vi "Code 0.0.5.vi"(0 "Value":refnum<k5>, 1 "status":bool, 2 "MaxSlide":dbl, 3 "File Path Control":path, 5 "Port":u16=8030, 7 "Connect Statut":refnum<vi>, 9 "Drv":u8(ring) items=["Drv 1", "Drv 2"], 11 "error in (no error)":errorcluster, 12 "Progress bar Value":refnum<vi>, 13 "String":refnum<vi>, 14 "Max":refnum<vi>) -> (4 "Error List":string, 6 "Status":bool, 15 "error out":errorcluster)   [LabVIEW 2017]
panel:
  out "Autobaud":bool
  in  "StopS.M. 2":bool
  in  "StopS.M.":bool
  in  "CatchNetworkFlag":bool
  in  "stop Listen":bool
  out "conn ID":refnum<k5>
  in  "Next Button":bool
  out "CheckSum":bool[][](array[boolean])
  out "CheckSum DataB":u16 format="%.0x"
  out "CheckSum Data":u16 format="%.0x"
  out "Writting Data":bool
  out "Send Header":bool
  out "sumHeader":u16 format="%.0x"
  # "Ver 0.0.7"
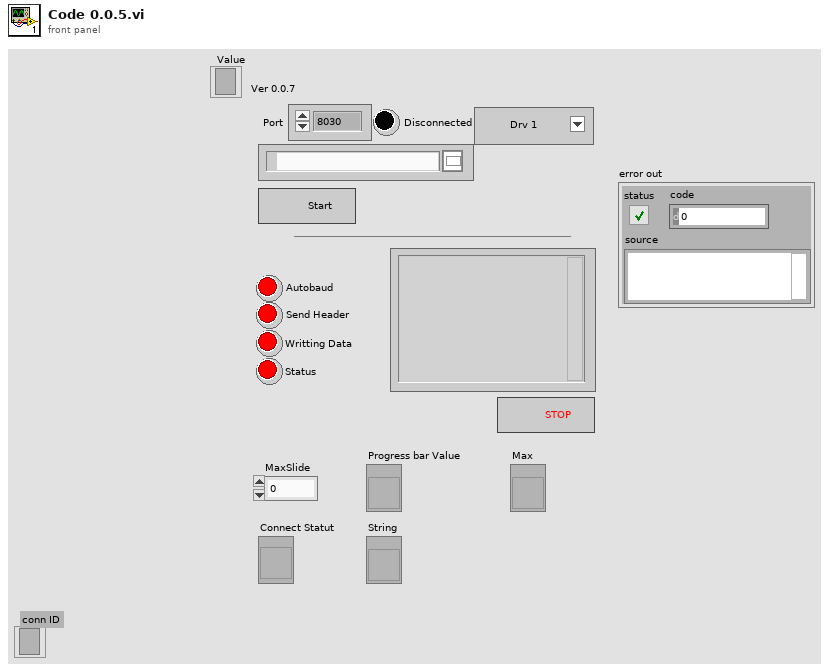
[diagram p1: front panel]
types:
  T1 = enum16{"open", "replace", "create", "open or create", "replace or create", "replace or create with confirmation"}
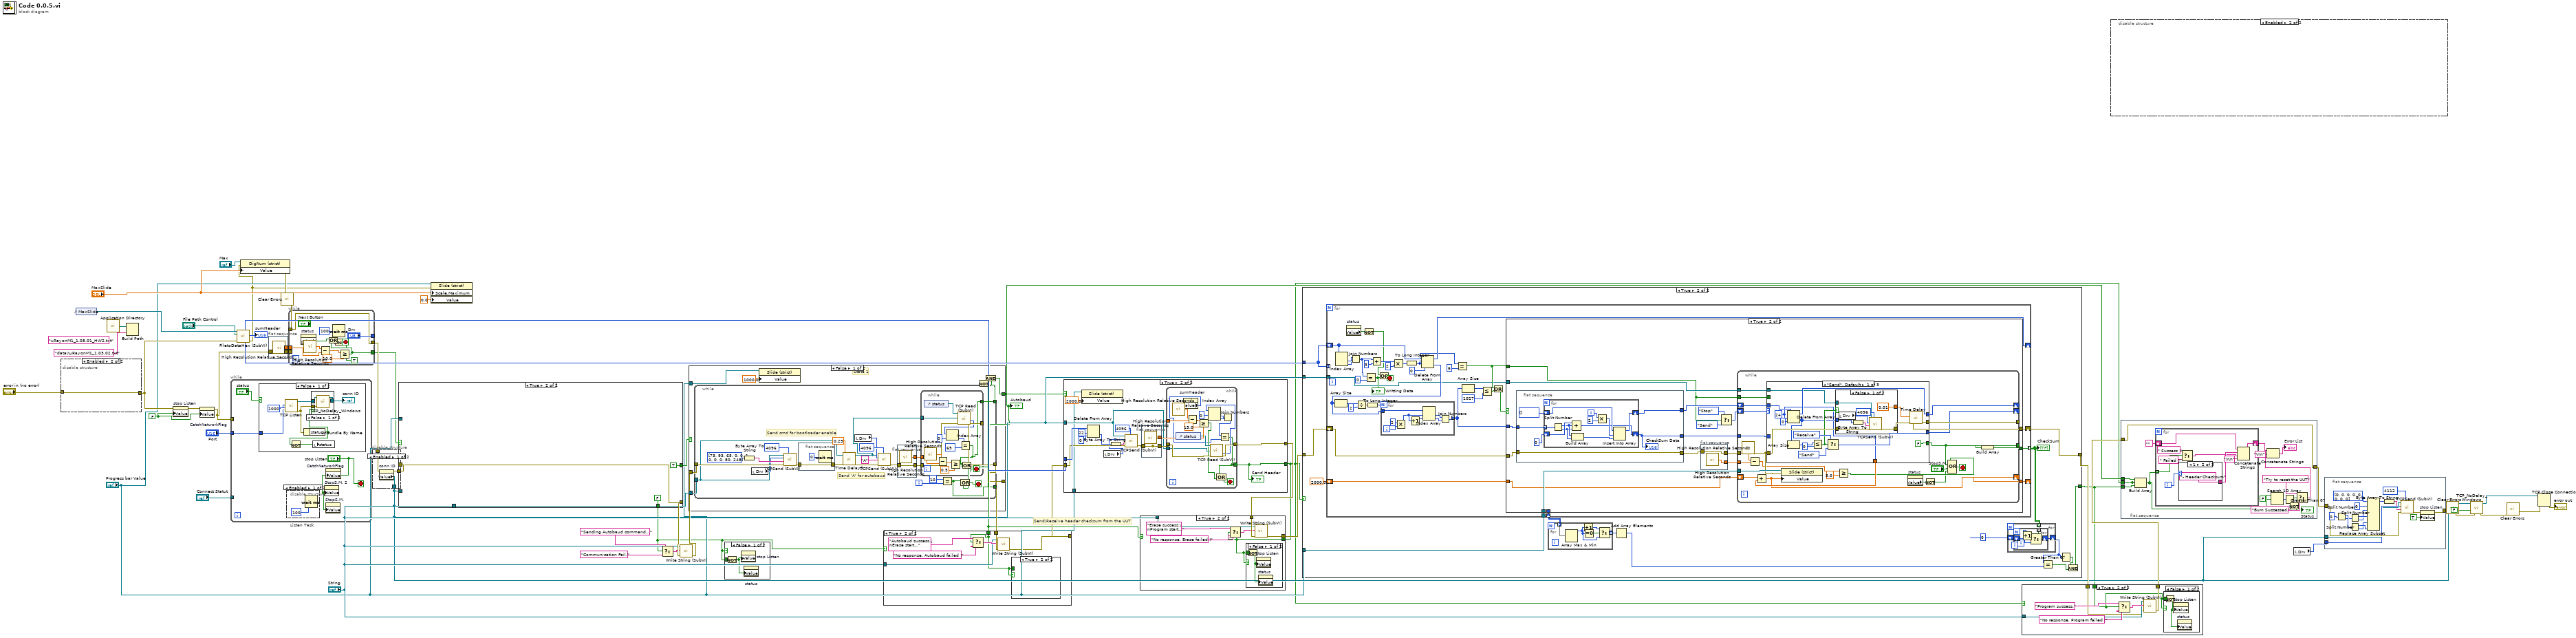
[diagram p0: block diagram]
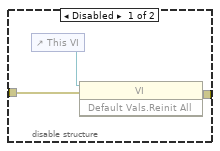
[diagram p2: hidden frame]
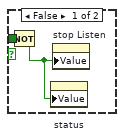
[diagram p7: hidden frame]
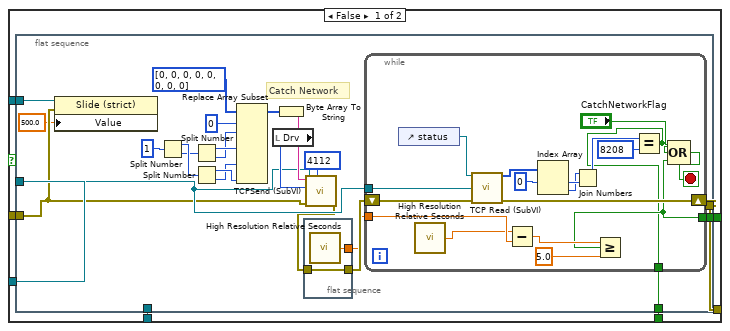
[diagram p10: hidden frame]
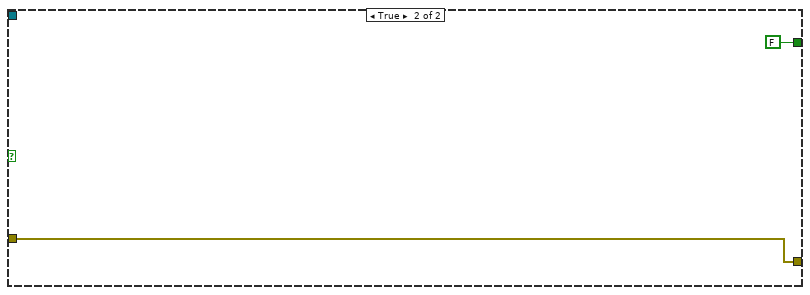
[diagram p11: hidden frame]
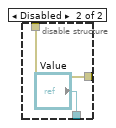
[diagram p12: hidden frame]
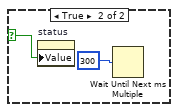
[diagram p15: hidden frame]
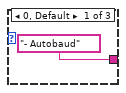
[diagram p16: hidden frame]
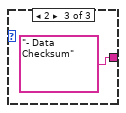
[diagram p17: hidden frame]
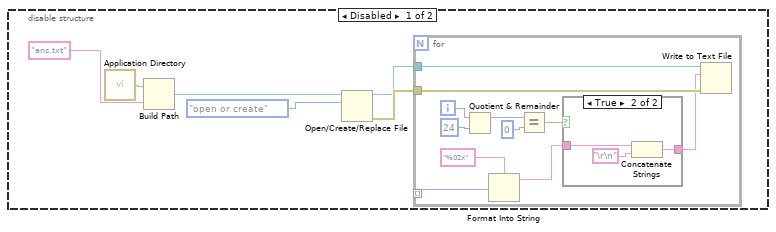
[diagram p18: hidden frame]
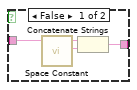
[diagram p19: hidden frame]
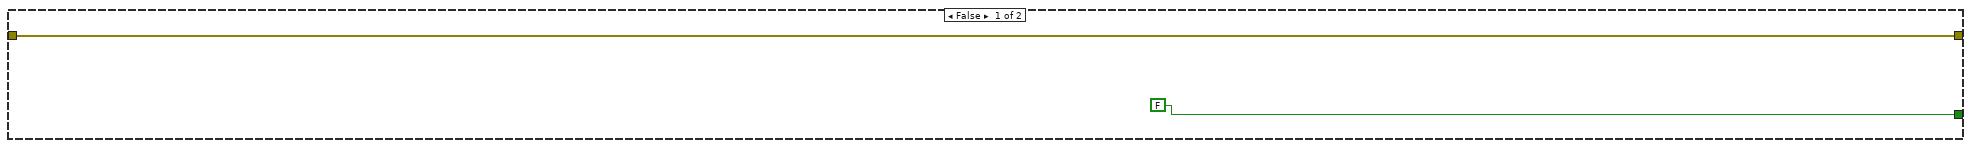
[diagram p20: hidden frame]
diagram:
  (unwired) "uRayonM1_1.05.01_HW2.txt" ("name or relative path")
  w40 = FALSE ("stop")
  # "Send/Receive header checksum from the UUT"
  n1 = disable-structure shown="Enabled" {
    disable-tunnel: "error in (no error)" -> [w56 w57]
    disable-tunnel: [w55 w57] -> w42
    frame Disabled {
      n2 = control-ref of="This VI"() -> (w54:refnum<vi>)
      n3 = invoke class="VI" method="Default Vals.Reinit All"(reference=w54, error in=w56) -> (error out=w55:errorcluster)  [unwired: 1 in, 2 out]
    }
    frame Enabled {
    }
  }
  n4 = control-ref of="MaxSlide"() -> (w39:refnum<vi>)
  n5 = call <vilib>:"Application Directory.vi"() -> ("Application Directory"=w47:path)
  n6 = Build Path(base path=w47, name or relative path="data\\uRayonM1_1.03.02.txt") -> ()  [unwired: 1 out]
  n7 = property on="stop Listen" class="Bool (strict)"(error in=w42, "Value"=w40) -> (error out=w41:errorcluster)  [unwired: 1 in, 1 out]
  n8 = property on="CatchNetworkFlag" class="Bool (strict)"(error in=w41, "Value"=w40) -> (error out=w6:errorcluster)  [unwired: 1 in, 1 out]
  n9 = while "Listen Task" {
    tunnel: w6 -> [_]
    tunnel: "Connect Statut" -> [_]
    tunnel: "Port" -> [w58]
    stop <- "stop Listen" stop-if-true
    n10 = case shown="False" "status" {
      selector: "status" -> [_ w73]
      tunnel: w58 -> [w62 _]
      frame False {
        n11 = call <vilib>:"TCP Listen.vi"("timeout ms (wait forever: -1)"=1000, "port"=w62) -> ("error out"=w66:errorcluster, "connection ID"=w65:refnum<k5>)  [unwired: 5 in, 3 out]
        n12 = Unbundle By Name(w66) -> ("status"=w64:bool)
        n13 = Not(x=w64) -> (.not. x?=w67:bool)
        n14 = case shown="False" w64 {
          tunnel: w66 -> [w71 _]
          tunnel: w65 -> [w70 w72]
          tunnel: [w69 w72] -> w63
          frame False {
            n15 = call "TCP_NoDelay_Windows.vi"("error in (no error)"=w71, "connID"=w70) -> ("connID 2"=w69:refnum<k5>)  [unwired: 4 in, 1 out]
          }
          frame True {
          }
        }
        "conn ID" <- w63
        n16 = local write "status"(w67) -> ()
      }
      frame True {
        n17 = property on="status" class="Bool (strict)"("Value"=w73) -> ()  [unwired: 2 in, 2 out]
        n18 = Wait Until Next ms Multiple(millisecond multiple=u32 300) -> ()  [unwired: 1 out]
      }
    }
    n19 = disable-structure shown="Enabled" {
      frame Enabled {
        n20 = Wait (ms)(milliseconds to wait=u32 100) -> ()  [unwired: 1 out]
      }
      frame Disabled {
      }
    }
    n21 = property on="StopS.M. 2" class="Bool (strict)"("Value"="stop Listen") -> ()  [unwired: 2 in, 2 out]
    n22 = property on="StopS.M." class="Bool (strict)"("Value"="stop Listen") -> ()  [unwired: 2 in, 2 out]
    n23 = property on="CatchNetworkFlag" class="Bool (strict)"("Value"="stop Listen") -> ()  [unwired: 2 in, 2 out]
  }
  n24 = call "FiletoDataHex (SubVI).vi"("error constant"=w42, "file path (use dialog)"="File Path Control", "Progress bar Max"=w39) -> ("error constant 2"=w12:errorcluster, "Array 2"=w53:u8[], "Array"=w51:u8[], "sumHeader"=→"sumHeader":u16)  [unwired: 2 in, 3 out]
  n25 = property class="DigNum (strict)"(reference="Max", error in=w12, "Value"="MaxSlide") -> (error out=w37:errorcluster)  [unwired: 1 out]
  n26 = flat-sequence {
    tunnel: [w76] -> w45
    tunnel: w6 -> [w75]
    tunnel: [w75] -> w5
    frame #0 {
      n27 = call <vilib>:"High Resolution Relative Seconds.vi"() -> ("relative seconds"=w76:dbl)
    }
  }
  n28 = call <vilib>:"Clear Errors.vi"("error in (no error)"=w37) -> ("error out"=w7:errorcluster)  [unwired: 5 in, 1 out]
  n29 = while {
    tunnel: w7 -> [w86]
    tunnel: ["Drv"] -> _
    tunnel: [w86] -> w44
    tunnel: w45 -> [w84]
    tunnel: [w79] -> w14
    tunnel: w5 -> [_]
    stop <- w78 stop-if-true
    n30 = property on="status" class="Bool (strict)"() -> ("Value"=w80:bool)  [unwired: 2 in, 2 out]
    n31 = call <vilib>:"High Resolution Relative Seconds.vi"() -> ("relative seconds"=w85:dbl)
    n32 = Subtract(x=w85, y=w84) -> (x-y=w83:dbl)
    n33 = Wait (ms)(milliseconds to wait=u32 100) -> ()  [unwired: 1 out]
    n34 = Greater Or Equal?(x=w83, y=10.0) -> (x >= y?=w79:bool)
    n35 = Or(x=w80, y=w79) -> (x .or. y?=w81:bool)
    n36 = And(x=w81, y=TRUE) -> (x .and. y?=w78:bool)
  }
  n37 = disable-structure shown="Enabled" {
    disable-tunnel: w44 -> [w91 w93]
    disable-tunnel: [w90 w93] -> w43
    disable-tunnel: [w89 "Value"] -> w18
    frame Enabled {
      n38 = property on="conn ID" class="Ref (strict)"(error in=w91) -> (error out=w90:errorcluster, "Value"=w89:refnum<k5>)  [unwired: 1 in, 1 out]
    }
    frame Disabled {
    }
  }
  n39 = case shown="True" w14 {
    tunnel: w43 -> [w100 w145]
    tunnel: [w99 TRUE] -> w33
    tunnel: [w98 w145] -> w31
    tunnel: [w97 FALSE] -> w9
    tunnel: "String" -> [w96 _]
    tunnel: w18 -> [w95 _]
    tunnel: "Progress bar Value" -> [w94 _]
    frame False {
      n40 = flat-sequence {
        tunnel: w95 -> [w109]
        tunnel: [w111] -> w98
        tunnel: w100 -> [w102]
        tunnel: [w108] -> w99
        tunnel: w96 -> [_]
        tunnel: [w104] -> w97
        tunnel: w94 -> [w103]
        frame #0 {
          # "Catch Network"
          n41 = property class="Slide (strict)"(reference=w103, error in=w102, "Value"=500.0) -> ()  [unwired: 2 out]
          n42 = Split Number(x=u32 1) -> (hi(x)=w121:u16, lo(x)=w120:u16)
          n43 = Split Number(x=w120) -> (hi(x)=w115:u8, lo(x)=w114:u8)
          n44 = Split Number(x=w121) -> (hi(x)=w113:u8, lo(x)=w112:u8)
          n45 = Replace Array Subset(array=u8[] [0, 0, 0, 0, 0, 0, 0, 0] ("unsigned byte array"), new element #1=w114, index #1=0 ("index"), new element #2=w115, new element #3=w112, new element #4=w113) -> (w116:u8[])  [unwired: 3 in]
          n46 = local read "Drv"() -> (w110:u8)
          n47 = Byte Array To String(unsigned byte array=w116) -> (string=w122:string)
          n48 = flat-sequence {
            tunnel: w107 -> [w125]
            tunnel: [w125] -> w106
            tunnel: [w124] -> w105
            frame #0 {
              n49 = call <vilib>:"High Resolution Relative Seconds.vi"() -> ("relative seconds"=w124:dbl)
            }
          }
          n50 = call "TCPSend (SubVI).vi"("Opcode"=u32 4112, "error in"=w102, "string"=w122, "Drv"=w110, "connection ID"=w109) -> ("error out"=w107:errorcluster)  [unwired: 6 in]
          n51 = while {
            shift-right: [w142] -> w111
            shift-left: w106 -> [w143]
            tunnel: w109 -> [w132]
            tunnel: [w127] -> w108
            tunnel: w105 -> [w131]
            tunnel: [w126] -> w104
            stop <- w138 stop-if-true
            n52 = control-ref of="status"() -> (w137:refnum<vi>)
            n53 = call <vilib>:"High Resolution Relative Seconds.vi"() -> ("relative seconds"=w130:dbl)
            n54 = call "TCP Read (SubVI).vi"("Status in"=w137, "Value"=w132, "error in (no error)"=w143) -> ("Rx data tmp"=w136:u8[], "error out"=w142:errorcluster)  [unwired: 2 in, 9 out]
            n55 = Subtract(x=w130, y=w131) -> (x-y=w129:dbl)
            n56 = Index Array(array=w136, index #1=0 ("index")) -> (element #1=w135:u8, element #2=w134:u8)  [unwired: 1 in]
            n57 = Join Numbers(hi=w134, lo=w135) -> ((hi.lo)=w141:u16)
            n58 = Greater Or Equal?(x=w129, y=5.0) -> (x >= y?=w127:bool)
            n59 = Equal?(x=w141, y=u16 8208) -> (x = y?=w126:bool)
            n60 = Compound Arithmetic op=OR("CatchNetworkFlag", w126, w127) -> (w138:bool)
          }
        }
      }
    }
    frame True {
    }
  }
  n61 = property class="Slide (strict)"(reference="Progress bar Value", error in=w12, "Scale.Maximum"="MaxSlide", "Value"=0.0) -> ()  [unwired: 2 out]
  n62 = Select(t="Sending Autobaud command...", s=w9, f="Communication Fail.") -> (s? t:f=w29:string)
  n63 = call "Write String (SubVI).vi"("error in (no error)"=w31, "string"=w29, "String in"="String") -> ("error out"=w30:errorcluster)  [unwired: 8 in]
  n64 = case shown="False" w33 {
    tunnel: w30 -> [w155 w197]
    tunnel: [w154 w197] -> w26
    tunnel: [w152 FALSE] -> w11
    tunnel: w18 -> [w153 _]
    tunnel: "Progress bar Value" -> [w148 _]
    frame False {
      # "State 1"
      n65 = while {
        tunnel: w155 -> [w172]
        tunnel: [w170] -> w154
        tunnel: w153 -> [w157]
        tunnel: [w160] -> w151
        tunnel: [w156] -> w150
        i -> [w176]
        stop <- w177 stop-if-true
        # "Send 'A' for autobaud"
        # "Send cmd for bootloader enable"
        n66 = Byte Array To String(unsigned byte array=u8[] [73, 93, 65, 0, 0, 1, 0, 0, 0, 80, 248] ("output array")) -> (string=w166:string)
        n67 = local read "Drv"() -> (w161:u8)
        n68 = call "TCPSend (SubVI).vi"("Opcode"=u32 4096, "error in"=w172, "string"=w166, "Drv"=w161, "connection ID"=w157) -> ("error out"=w168:errorcluster)  [unwired: 6 in]
        n69 = flat-sequence {
          tunnel: w168 -> [w178]
          tunnel: [w178] -> w167
          frame #0 {
            n70 = Wait (ms)(milliseconds to wait=u32 0) -> ()  [unwired: 1 out]
          }
        }
        n71 = call "Time Delay3"("error in (no error)"=w167, "Delay Time (s)"=0.25) -> ("error out"=w159:errorcluster)  [unwired: 9 in]
        n72 = local read "Drv"() -> (w162:u8)
        n73 = call "TCPSend (SubVI).vi"("Opcode"=u32 4096, "error in"=w159, "string"="A" ("write buffer"), "Drv"=w162, "connection ID"=w157) -> ("error out"=w171:errorcluster)  [unwired: 6 in]
        n74 = flat-sequence {
          tunnel: w171 -> [w181]
          tunnel: [w181] -> w174
          tunnel: [w180] -> w173
          frame #0 {
            n75 = call <vilib>:"High Resolution Relative Seconds.vi"() -> ("relative seconds"=w180:dbl)
          }
        }
        n76 = while {
          tunnel: w174 -> [w186]
          tunnel: w173 -> [w192]
          tunnel: [w185] -> w170
          tunnel: [w183] -> w160
          tunnel: w157 -> [w182]
          stop <- w184 stop-if-true
          n77 = control-ref of="status"() -> (w196:refnum<vi>)
          n78 = call <vilib>:"High Resolution Relative Seconds.vi"() -> ("relative seconds"=w193:dbl)
          n79 = Subtract(x=w193, y=w192) -> (x-y=w191:dbl)
          n80 = Greater Or Equal?(x=w191, y=0.5) -> (x >= y?=w189:bool)
          n81 = call "TCP Read (SubVI).vi"("Status in"=w196, "Value"=w182, "error in (no error)"=w186) -> ("Drv Array"=w194:u8[], "error out"=w185:errorcluster)  [unwired: 2 in, 9 out]
          n82 = Index Array(array=w194, index=0) -> (element=w188:u8)
          n83 = Equal?(x=w188, y=u8 65) -> (x = y?=w183:bool)
          n84 = Or(x=w183, y=w189) -> (x .or. y?=w184:bool)
        }
        n85 = Equal?(x=10, y=w176) -> (x = y?=w156:bool)
        n86 = Compound Arithmetic op=OR(w156, w160) -> (w177:bool)
      }
      n87 = property class="Slide (strict)"(reference=w148, "Value"=1000.0) -> ()  [unwired: 1 in, 2 out]
      n88 = Not(x=w150) -> (.not. x?=w149:bool)
      n89 = And(x=w151, y=w149) -> (x .and. y?=w152:bool)
    }
    frame True {
    }
  }
  "Autobaud" <- w11
  n90 = case shown="False" w9 {
    tunnel: w9 -> [w200 _]
    frame False {
      n91 = Not(x=w200) -> (.not. x?=w199:bool)
      n92 = property on="stop Listen" class="Bool (strict)"("Value"=w199) -> ()  [unwired: 2 in, 2 out]
      n93 = property on="status" class="Bool (strict)"("Value"=w199) -> ()  [unwired: 2 in, 2 out]
    }
    frame True {
    }
  }
  n94 = case shown="True" w9 {
    tunnel: w26 -> [w201 w208]
    tunnel: [w201 w207] -> w25
    tunnel: "String" -> [_ w203]
    tunnel: w11 -> [_ w202]
    frame False {
    }
    frame True {
      n95 = Select(t="Autobaud success.\nErase start...", s=w202, f="No response, Autobaud failed !") -> (s? t:f=w206:string)
      n96 = call "Write String (SubVI).vi"("error in (no error)"=w208, "string"=w206, "String in"=w203) -> ("error out"=w207:errorcluster)  [unwired: 8 in]
      n97 = case shown="True" w202 {
        tunnel: w202 -> [w210 _]
        frame False {
          n98 = Not(x=w210) -> (.not. x?=w209:bool)
          n99 = property on="status" class="Bool (strict)"("Value"=w209) -> ()  [unwired: 2 in, 2 out]
          n100 = property on="stop Listen" class="Bool (strict)"("Value"=w209) -> ()  [unwired: 2 in, 2 out]
        }
        frame True {
        }
      }
    }
  }
  n101 = case shown="True" w11 {
    tunnel: w25 -> [w212 w226]
    tunnel: [w212 w228] -> w24
    tunnel: w51 -> [_ w227]
    tunnel: [FALSE w217] -> w10
    tunnel: w18 -> [_ w215]
    tunnel: "Progress bar Value" -> [_ w214]
    frame False {
    }
    frame True {
      n102 = property class="Slide (strict)"(reference=w214, "Value"=2000.0) -> ()  [unwired: 1 in, 2 out]
      n103 = Delete From Array(array=w227, length=22, index=0) -> (deleted portion=w222:u8[])  [unwired: 1 out]
      n104 = local read "Drv"() -> (w216:u8)
      n105 = Byte Array To String(unsigned byte array=w222) -> (string=w220:string)
      n106 = call "TCPSend (SubVI).vi"("Opcode"=u32 4096, "error in"=w226, "string"=w220, "Drv"=w216, "connection ID"=w215) -> ("error out"=w225:errorcluster)  [unwired: 6 in]
      n107 = flat-sequence {
        tunnel: w225 -> [w229]
        tunnel: [w229] -> _
        tunnel: [w230] -> w218
        tunnel: [w229] -> w219
        frame #0 {
          n108 = call <vilib>:"High Resolution Relative Seconds.vi"() -> ("relative seconds"=w230:dbl)
        }
      }
      n109 = while {
        tunnel: w219 -> [w242]
        tunnel: [w241] -> w228
        tunnel: w218 -> [w246]
        tunnel: [w232] -> w217
        tunnel: w215 -> [w231]
        stop <- w238 stop-if-true
        n110 = call <vilib>:"High Resolution Relative Seconds.vi"() -> ("relative seconds"=w247:dbl)
        n111 = control-ref of="status"() -> (w243:refnum<vi>)
        n112 = property on="sumHeader" class="DigNum (strict)"() -> ("Value"=w233:u16)  [unwired: 2 in, 2 out]
        n113 = Subtract(x=w247, y=w246) -> (x-y=w245:dbl)
        n114 = Greater Or Equal?(x=w245, y=15.0) -> (x >= y?=w237:bool)
        n115 = call "TCP Read (SubVI).vi"("Status in"=w243, "Value"=w231, "error in (no error)"=w242) -> ("Drv Array"=w239:u8[], "error out"=w241:errorcluster)  [unwired: 2 in, 9 out]
        n116 = Index Array(array=w239, index #1=0 ("index")) -> (element #1=w235:u8, element #2=w236:u8)  [unwired: 1 in]
        n117 = Join Numbers(hi=w236, lo=w235) -> ((hi.lo)=w234:u16)
        n118 = Equal?(x=w234, y=w233) -> (x = y?=w232:bool)
        n119 = Compound Arithmetic op=OR(w232, w237) -> (w238:bool)
      }
      "Send Header" <- w217
    }
  }
  n120 = case shown="True" w11 {
    tunnel: w24 -> [w248 w255]
    tunnel: [w248 w254] -> w23
    tunnel: "String" -> [_ w250]
    tunnel: w10 -> [_ w249]
    frame False {
    }
    frame True {
      n121 = Select(t="Erase success.\nProgram start...", s=w249, f="No response, Erase failed !") -> (s? t:f=w251:string)
      n122 = case shown="False" w249 {
        tunnel: w249 -> [w257 _]
        frame False {
          n123 = Not(x=w257) -> (.not. x?=w256:bool)
          n124 = property on="stop Listen" class="Bool (strict)"("Value"=w256) -> ()  [unwired: 2 in, 2 out]
          n125 = property on="status" class="Bool (strict)"("Value"=w256) -> ()  [unwired: 2 in, 2 out]
        }
        frame True {
        }
      }
      n126 = call "Write String (SubVI).vi"("error in (no error)"=w255, "string"=w251, "String in"=w250) -> ("error out"=w254:errorcluster)  [unwired: 8 in]
    }
  }
  n127 = case shown="True" w10 {
    tunnel: w23 -> [w258 w273]
    tunnel: [w258 w272] -> w21
    tunnel: w53 -> [_ w274]
    tunnel: [FALSE w263] -> w13
    tunnel: w18 -> [_ w262]
    tunnel: "Progress bar Value" -> [_ w261]
    frame False {
    }
    frame True {
      n128 = for {
        shift-right: [w312] -> _
        shift-left: w274 -> [w322]
        tunnel: w274 -> [_] mode=indexing
        tunnel: [w301] -> w269 mode=indexing
        shift-right: [w295] -> w272
        shift-left: w273 -> [w296]
        tunnel: [w294] -> w271 mode=indexing
        tunnel: w262 -> [w293]
        shift-right: [w291] -> _
        shift-left: 2000.0 -> [w292]
        tunnel: w261 -> [w290]
        stop <- w289 stop-if-true
        n129 = Index Array(array=w322) -> (element #1=w321:u8, element #2=w320:u8)  [unwired: 2 in]
        n130 = property on="status" class="Bool (strict)"() -> ("Value"=w288:bool)  [unwired: 2 in, 2 out]
        n131 = Join Numbers(hi=w320, lo=w321) -> ((hi.lo)=w298:u16)
        n132 = Not(x=w288) -> (.not. x?=w287:bool)
        n133 = Equal?(x=w298, y=u16 0) -> (x = y?=w315:bool)
        "Writting Data" <- w315
        n134 = Add(x=w298, y=u32 3) -> (x+y=w318:u32)
        n135 = Or(x=w287, y=w315) -> (x .or. y?=w289:bool)
        n136 = Multiply(x=w318, y=u32 2) -> (x*y=w316:u32)
        n137 = To Long Integer(number=w316) -> (32bit integer=w299:i32)
        n138 = Delete From Array(array=w322, length=w299, index=0) -> (deleted portion=w300:u8[], array with subset deleted=w312:u8[])
        n139 = Array Size(array=w300) -> (size(s)=w309:i32)
        n140 = Divide(x=w309, y=2) -> (x/y=w311:dbl)
        n141 = To Long Integer(number=w311) -> (32bit integer=w308:i32)
        n142 = for {
          N: w308 -> [_]
          tunnel: w300 -> [w590]
          tunnel: [w586] -> w305 mode=indexing
          i -> [w589]
          n143 = Multiply(x=2, y=w589) -> (x*y=w592:i32)
          n144 = Increment(x=w592) -> (x+1=w593:i32)
          n145 = Index Array(array=w590, index #1=w592, index #2=w593) -> (element #1=w588:u8, element #2=w587:u8)
          n146 = Join Numbers(hi=w588, lo=w587) -> ((hi.lo)=w586:u16)
        }
        n147 = Equal?(x=w299, y=6) -> (x = y?=w297:bool)
        n148 = Array Size(array=w305) -> (size(s)=w307:i32)
        n149 = Less Or Equal?(x=w307, y=1027) -> (x <= y?=w303:bool)
        n150 = Or(x=w297, y=w303) -> (x .or. y?=w302:bool)
        n151 = case shown="True" w302 {
          tunnel: w296 -> [w330 w480]
          tunnel: [w331 w478] -> w295
          tunnel: w305 -> [w328 w482]
          tunnel: [w329 w481] -> w301
          tunnel: w297 -> [_ w465]
          tunnel: [w327 _] -> w294
          tunnel: w293 -> [w326 w472]
          tunnel: w292 -> [w325 w470]
          tunnel: [w323 w469] -> w291
          tunnel: w290 -> [w324 w471]
          frame False {
            n152 = while {
              tunnel: w328 -> [_]
              tunnel: [w342] -> w329 mode=indexing
              shift-right: [w355] -> w331
              shift-left: w330 -> [w343]
              shift-right: [w348] -> _
              shift-left: w328 -> [w354]
              tunnel: [w340] -> w327 mode=indexing
              tunnel: w326 -> [w339]
              tunnel: w324 -> [w337]
              shift-right: [w336] -> w323
              shift-left: w325 -> [w338]
              i -> [w340]
              stop <- w335 stop-if-true
              n153 = Equal To 0?(x=w340) -> (x = 0?=w347:bool)
              n154 = Select(t=1027 ("length"), s=w347, f=1024 ("length")) -> (s? t:f=w344:i32)
              n155 = Delete From Array(array=w354, length=w344, index=0) -> (deleted portion=w341:u16[], array with subset deleted=w348:u16[])
              n156 = Array Size(array=w341) -> (size(s)=w352:i32)
              n157 = Greater?(x=w352, y=1) -> (0:w350:bool)
              n158 = Not(x=w350) -> (.not. x?=w349:bool)
              n159 = case shown="True" w350 {
                tunnel: [w359 w371] -> w355
                tunnel: w343 -> [w359 w373]
                tunnel: [FALSE w369] -> w342
                tunnel: w341 -> [_ w374]
                tunnel: w339 -> [_ w367]
                tunnel: w338 -> [w357 w365]
                tunnel: [w357 w364] -> w336
                tunnel: w337 -> [_ w366]
                tunnel: [TRUE ("Time has Elapsed") w363] -> w334
                frame False {
                }
                frame True {
                  n160 = flat-sequence {
                    tunnel: w373 -> [w449]
                    tunnel: [w451] -> w368
                    tunnel: [w448] -> w370
                    tunnel: w374 -> [w450]
                    tunnel: [w449] -> w362
                    frame #0 {
                      n161 = for {
                        tunnel: w450 -> [w464] mode=indexing
                        shift-right: [w459] -> w451
                        shift-left: u8[] [] -> [w458]
                        shift-right: [w456] -> w448
                        shift-left: u16 0 -> [w457]
                        i -> [w463]
                        n162 = Split Number(x=w464) -> (hi(x)=w455:u8, lo(x)=w454:u8)
                        n163 = Build Array(w455, w454) -> (w461:u8[])
                        n164 = Compound Arithmetic op=ADD(w457, w455, w454) -> (w456:u16)
                        n165 = Multiply(x=w463, y=2) -> (x*y=w460:i32)
                        n166 = Insert Into Array(array=w458, index=w460, new element=w461) -> (w459:u8[])
                      }
                      "CheckSum DataB" <- w448
                    }
                  }
                  n167 = flat-sequence {
                    tunnel: w362 -> [w376]
                    tunnel: [w376] -> w361
                    tunnel: [w375] -> w360
                    frame #0 {
                      n168 = call <vilib>:"High Resolution Relative Seconds.vi"() -> ("relative seconds"=w375:dbl)
                    }
                  }
                  n169 = while {
                    shift-right: [w396] -> _
                    shift-left: enum16{"Stop", "Receive", "Send"}."Send" -> [w398]
                    shift-right: [w394] -> _
                    shift-left: w368 -> [w397]
                    tunnel: w370 -> [w395]
                    tunnel: [w390] -> w369
                    tunnel: [w393] -> w371
                    tunnel: w367 -> [w389]
                    tunnel: w366 -> [w388]
                    shift-right: [w385] -> w364
                    shift-left: w365 -> [w387]
                    tunnel: [w379] -> w363
                    tunnel: w361 -> [w384]
                    tunnel: w360 -> [w383]
                    stop <- w392 stop-if-true
                    n170 = call <vilib>:"High Resolution Relative Seconds.vi"() -> ("relative seconds"=w382:dbl)
                    n171 = Subtract(x=w382, y=w383) -> (x-y=w381:dbl)
                    n172 = case shown="\"Send\", Default" w398 {
                      selector: w398 -> [_ _ w447]
                      tunnel: w397 -> [w414 w432 w445]
                      tunnel: [w411 w434 w447] -> w396
                      tunnel: w384 -> [w410 w430 w444]
                      tunnel: w395 -> [_ w436 _]
                      tunnel: [FALSE FALSE TRUE] -> w390
                      tunnel: [w406 w432 w445] -> w394
                      tunnel: [w404 w431 w444] -> w393
                      tunnel: w389 -> [w400 w427 _]
                      tunnel: [w399 0.0 ("y") 0.0 ("y")] -> w386
                      frame "Send", Default {
                        w399 = 64 ("length")
                        n173 = Delete From Array(array=w414, length=w399, index=0) -> (deleted portion=w403:u8[], array with subset deleted=w406:u8[])
                        n174 = Array Size(array=w403) -> (size(s)=w412:i32)
                        n175 = Less Or Equal?(x=w412, y=0) -> (x <= y?=w402:bool)
                        n176 = case shown="False" w402 {
                          tunnel: w403 -> [w420 _]
                          tunnel: w410 -> [w419 w425]
                          tunnel: [w418 w425] -> w405
                          tunnel: [0.01 ("Delay Time (s)") 0.0 ("Delay Time (s)")] -> w401
                          tunnel: w400 -> [w416 _]
                          frame False {
                            n177 = local read "Drv"() -> (w421:u8)
                            n178 = Byte Array To String(unsigned byte array=w420) -> (string=w422:string)
                            n179 = call "TCPSend (SubVI).vi"("Opcode"=u32 4096, "error in"=w419, "string"=w422, "Drv"=w421, "connection ID"=w416) -> ("error out"=w418:errorcluster)  [unwired: 6 in]
                          }
                          frame True {
                          }
                        }
                        n180 = Select(t=enum16{"Stop", "Receive", "Send"}."Receive", s=w402, f=enum16{"Stop", "Receive", "Send"}."Send") -> (s? t:f=w411:enum16{"Stop", "Receive", "Send"})
                        n181 = call "Time Delay2"("error in (no error)"=w405, "Delay Time (s)"=w401) -> ("error out"=w404:errorcluster)  [unwired: 9 in]
                      }
                      frame "Receive" {
                        n182 = control-ref of="status"() -> (w442:refnum<vi>)
                        n183 = call "TCP Read (SubVI).vi"("Status in"=w442, "Value"=w427, "error in (no error)"=w430) -> ("Drv Array"=w438:u8[], "error out"=w431:errorcluster)  [unwired: 2 in, 9 out]
                        n184 = Index Array(array=w438, index #1=0 ("index")) -> (element #1=w441:u8, element #2=w440:u8)  [unwired: 1 in]
                        n185 = Join Numbers(hi=w440, lo=w441) -> ((hi.lo)=w437:u16)
                        n186 = Equal?(x=w437, y=w436) -> (x = y?=w429:bool)
                        n187 = Select(t=enum16{"Stop", "Receive", "Send"}."Stop", s=w429, f=enum16{"Stop", "Receive", "Send"}."Receive") -> (s? t:f=w434:enum16{"Stop", "Receive", "Send"})
                      }
                      frame "Stop" {
                      }
                    }
                    n188 = Add(x=w387, y=w386) -> (x+y=w385:dbl)
                    n189 = Greater Or Equal?(x=w381, y=5.0) -> (x >= y?=w379:bool)
                    n190 = property class="Slide (strict)"(reference=w388, error in=w384, "Value"=w385) -> ()  [unwired: 2 out]
                    n191 = property on="status" class="Bool (strict)"() -> ("Value"=w378:bool)  [unwired: 2 in, 2 out]
                    n192 = Not(x=w378) -> (.not. x?=w377:bool)
                    n193 = Compound Arithmetic op=OR(w390, "StopS.M. 2", w379, w377) -> (w392:bool)
                  }
                }
              }
              n194 = property on="status" class="Bool (strict)"() -> ("Value"=w333:bool)  [unwired: 2 in, 2 out]
              n195 = Not(x=w333) -> (.not. x?=w332:bool)
              n196 = Compound Arithmetic op=OR(w334, w349, w332) -> (w335:bool)
            }
          }
          frame True {
            n197 = flat-sequence {
              tunnel: w480 -> [w570]
              tunnel: [w572] -> w473
              tunnel: w482 -> [w571]
              tunnel: [w570] -> w468
              tunnel: [w569] -> w479
              frame #0 {
                n198 = for {
                  tunnel: w571 -> [w585] mode=indexing
                  shift-right: [w580] -> w572
                  shift-left: u8[] [] -> [w579]
                  shift-right: [w577] -> w569
                  shift-left: u16 0 -> [w578]
                  i -> [w584]
                  n199 = Split Number(x=w585) -> (hi(x)=w576:u8, lo(x)=w575:u8)
                  n200 = Build Array(w576, w575) -> (w582:u8[])
                  n201 = Compound Arithmetic op=ADD(w578, w576, w575) -> (w577:u16)
                  n202 = Multiply(x=w584, y=2) -> (x*y=w581:i32)
                  n203 = Insert Into Array(array=w579, index=w581, new element=w582) -> (w580:u8[])
                }
                "CheckSum Data" <- w569
              }
            }
            n204 = flat-sequence {
              tunnel: w468 -> [w484]
              tunnel: [w484] -> w467
              tunnel: [w483] -> w466
              frame #0 {
                n205 = call <vilib>:"High Resolution Relative Seconds.vi"() -> ("relative seconds"=w483:dbl)
              }
            }
            n206 = Select(t=enum16{"Stop", "Receive", "Send"}."Stop", s=w465, f=enum16{"Stop", "Receive", "Send"}."Send") -> (s? t:f=w476:enum16{"Stop", "Receive", "Send"})
            n207 = while {
              shift-right: [w505] -> _
              shift-left: w476 -> [w507]
              shift-right: [w503] -> _
              shift-left: w473 -> [w506]
              tunnel: w467 -> [w495]
              tunnel: w479 -> [w504]
              tunnel: [w502] -> w474
              tunnel: [w501] -> w478
              tunnel: w472 -> [w498]
              tunnel: w471 -> [w497]
              shift-right: [w493] -> w469
              shift-left: w470 -> [w496]
              tunnel: w466 -> [w492]
              tunnel: w465 -> [w487]
              stop <- w500 stop-if-true
              n208 = call <vilib>:"High Resolution Relative Seconds.vi"() -> ("relative seconds"=w491:dbl)
              n209 = Subtract(x=w491, y=w492) -> (x-y=w490:dbl)
              n210 = case shown="\"Send\", Default" w507 {
                selector: w507 -> [_ _ w561]
                tunnel: w506 -> [w523 w540 w552]
                tunnel: [w520 w542 w561] -> w505
                tunnel: w495 -> [w519 w538 w556]
                tunnel: w504 -> [_ w545 _]
                tunnel: [FALSE FALSE TRUE] -> w502
                tunnel: [w515 w540 w552] -> w503
                tunnel: [w513 w539 w555] -> w501
                tunnel: w498 -> [w509 w536 w557]
                tunnel: [w508 0.0 ("x") 0.0 ("x")] -> w494
                tunnel: w487 -> [_ _ w554]
                frame "Send", Default {
                  w508 = 24 ("length")
                  n211 = Delete From Array(array=w523, length=w508, index=0) -> (deleted portion=w511:u8[], array with subset deleted=w515:u8[])
                  n212 = Array Size(array=w511) -> (size(s)=w521:i32)
                  n213 = Less Or Equal?(x=w521, y=0) -> (x <= y?=w512:bool)
                  n214 = Select(t=enum16{"Stop", "Receive", "Send"}."Receive", s=w512, f=enum16{"Stop", "Receive", "Send"}."Send") -> (s? t:f=w520:enum16{"Stop", "Receive", "Send"})
                  n215 = case shown="False" w512 {
                    tunnel: w511 -> [w529 _]
                    tunnel: w519 -> [w528 w534]
                    tunnel: [w527 w534] -> w514
                    tunnel: [0.01 ("Delay Time (s)") 0.0 ("Delay Time (s)")] -> w510
                    tunnel: w509 -> [w525 _]
                    frame False {
                      n216 = local read "Drv"() -> (w530:u8)
                      n217 = Byte Array To String(unsigned byte array=w529) -> (string=w531:string)
                      n218 = call "TCPSend (SubVI).vi"("Opcode"=u32 4096, "error in"=w528, "string"=w531, "Drv"=w530, "connection ID"=w525) -> ("error out"=w527:errorcluster)  [unwired: 6 in]
                    }
                    frame True {
                    }
                  }
                  n219 = call "Time Delay"("error in (no error)"=w514, "Delay Time (s)"=w510) -> ("error out"=w513:errorcluster)  [unwired: 9 in]
                }
                frame "Receive" {
                  n220 = control-ref of="status"() -> (w551:refnum<vi>)
                  n221 = call "TCP Read (SubVI).vi"("Status in"=w551, "Value"=w536, "error in (no error)"=w538) -> ("Drv Array"=w547:u8[], "error out"=w539:errorcluster)  [unwired: 2 in, 9 out]
                  n222 = Index Array(array=w547, index #1=0 ("index")) -> (element #1=w550:u8, element #2=w549:u8)  [unwired: 1 in]
                  n223 = Join Numbers(hi=w549, lo=w550) -> ((hi.lo)=w546:u16)
                  n224 = Equal?(x=w546, y=w545) -> (x = y?=w544:bool)
                  n225 = Select(t=enum16{"Stop", "Receive", "Send"}."Stop", s=w544, f=enum16{"Stop", "Receive", "Send"}."Receive") -> (s? t:f=w542:enum16{"Stop", "Receive", "Send"})
                }
                frame "Stop" {
                  n226 = local read "Drv"() -> (w553:u8)
                  n227 = Byte Array To String(unsigned byte array=w552) -> (string=w558:string)
                  n228 = case shown="True" w554 {
                    tunnel: w558 -> [_ w568]
                    tunnel: w556 -> [w562 w566]
                    tunnel: [w562 w565] -> w555
                    tunnel: w557 -> [_ w564]
                    tunnel: w553 -> [_ w563]
                    frame False {
                    }
                    frame True {
                      n229 = call "TCPSend (SubVI).vi"("Opcode"=u32 4096, "error in"=w566, "string"=w568, "Drv"=w563, "connection ID"=w564) -> ("error out"=w565:errorcluster)  [unwired: 6 in]
                    }
                  }
                }
              }
              n230 = Add(x=w496, y=w494) -> (x+y=w493:dbl)
              n231 = property class="Slide (strict)"(reference=w497, error in=w495, "Value"=w493) -> ()  [unwired: 2 out]
              n232 = Greater Or Equal?(x=w490, y=5.0) -> (x >= y?=w488:bool)
              n233 = property on="status" class="Bool (strict)"() -> ("Value"=w486:bool)  [unwired: 2 in, 2 out]
              n234 = Not(x=w486) -> (.not. x?=w485:bool)
              n235 = Compound Arithmetic op=OR(w488, w502, "StopS.M.", w485) -> (w500:bool)
            }
            n236 = Build Array(w474) -> (w481:bool[])
          }
        }
      }
      "CheckSum" <- w269
      n237 = for {
        tunnel: w271 -> [w286] mode=indexing
        tunnel: [w282] -> w270 mode=indexing
        n238 = Array Max & Min(array=w286) -> (max value=w283:i32)  [unwired: 3 out]
        n239 = Increment(x=w283) -> (x+1=w284:i32)
        n240 = Equal To 0?(x=w283) -> (x = 0?=w285:bool)
        n241 = Select(t=w284, s=w285, f=w283) -> (s? t:f=w282:i32)
      }
      n242 = Add Array Elements(numeric array=w270) -> (sum=w267:i32)
      n243 = for {
        tunnel: w269 -> [w277] mode=indexing
        shift-right: [w276] -> w266
        shift-left: 0 -> [w275]
        n244 = for {
          tunnel: w277 -> [w281] mode=indexing
          shift-right: [w279] -> w276
          shift-left: w275 -> [w278]
          n245 = Increment(x=w278) -> (x+1=w280:i32)
          n246 = Select(t=w280, s=w281, f=w278) -> (s? t:f=w279:i32)
        }
      }
      n247 = Equal?(x=w266, y=w267) -> (x = y?=w264:bool)
      n248 = Greater Than 0?(x=w266) -> (x > 0?=w265:bool)
      n249 = And(x=w265, y=w264) -> (x .and. y?=w263:bool)
    }
  }
  n250 = case shown="True" w10 {
    tunnel: "String" -> [_ w598]
    tunnel: w21 -> [w594 w597]
    tunnel: [w594 w596] -> w20
    tunnel: w13 -> [_ w595]
    frame False {
    }
    frame True {
      n251 = Select(t="Program success.", s=w595, f="No response, Program failed !") -> (s? t:f=w601:string)
      n252 = call "Write String (SubVI).vi"("error in (no error)"=w597, "string"=w601, "String in"=w598) -> ("error out"=w596:errorcluster)  [unwired: 8 in]
      n253 = case shown="False" w595 {
        tunnel: w595 -> [w603 _]
        frame False {
          n254 = Not(x=w603) -> (.not. x?=w602:bool)
          n255 = property on="stop Listen" class="Bool (strict)"("Value"=w602) -> ()  [unwired: 2 in, 2 out]
          n256 = property on="status" class="Bool (strict)"("Value"=w602) -> ()  [unwired: 2 in, 2 out]
        }
        frame True {
        }
      }
    }
  }
  n257 = disable-structure shown="Enabled" {
    frame Disabled {
      n258 = call <vilib>:"Application Directory.vi"() -> ("Application Directory"=w608:path)
      n259 = Build Path(base path=w608, name or relative path="ans.txt") -> (appended path=w607:path)
      n260 = Open/Create/Replace File(file path (use dialog)=w607, operation (0:open)=T1."open or create") -> (refnum out=w604:refnum<file>, error out=w605:errorcluster)  [unwired: 4 in, 1 out]
      n261 = for {
        tunnel: _ -> [w620] mode=indexing
        tunnel: w605 -> [w618]
        tunnel: w604 -> [w617]
        i -> [w613]
        n262 = Quotient & Remainder(x=w613, y=24 ("x")) -> (x-y*floor(x/y)=w611:i32)  [unwired: 1 out]
        n263 = Format Into String(format string="%02x", w620) -> (resulting string=w616:string)  [unwired: 2 in, 1 out]
        n264 = Equal?(x=w611, y=0) -> (x = y?=w614:bool)
        n265 = case shown="True" w614 {
          tunnel: w616 -> [w623 w626]
          tunnel: [w622 w625] -> w615
          frame False {
            n266 = call <vilib>:"Space Constant.vi"() -> ("String"=w621:string)
            n267 = Concatenate Strings(w623, w621) -> (w622:string)
          }
          frame True {
            n268 = Concatenate Strings(w626, "\r\n") -> (w625:string)
          }
        }
        n269 = Write to Text File(file (use dialog)=w617, text=w615, error in=w618) -> ()  [unwired: 1 in, 3 out]
      }
    }
    frame Enabled {
    }
  }
  n270 = flat-sequence {
    tunnel: w20 -> [w642]
    tunnel: [w642] -> w50
    tunnel: w11 -> [w641]
    tunnel: [w629] -> _
    tunnel: w13 -> [w640]
    tunnel: w10 -> [w629]
    frame #0 {
      n271 = Build Array(w641, w629, w640) -> (w635:bool[])
      n272 = for {
        tunnel: w635 -> [w651] mode=indexing
        shift-right: [w649] -> w638
        shift-left: "" -> [w650]
        i -> [w647]
        n273 = case shown="1" w647 {
          tunnel: ["- Autobaud" "- Header Checksum" "- Data Checksum"] -> w646
          frame 0, Default {
          }
          frame 1 {
          }
          frame 2 {
          }
        }
        n274 = Select(t=" Success !", s=w651, f=" Failed !") -> (s? t:f=w645:string)
        n275 = Concatenate Strings(w650, w646, w645, "\r\n") -> (w649:string)
      }
      n276 = Search 1D Array(1D array=w635, element=FALSE) -> (index of element=w633:i32)  [unwired: 1 in]
      n277 = Greater Than 0?(x=w633) -> (x > 0?=w628:bool)
      n278 = Not(x=w628) -> (.not. x?=→"Status":bool)
      n279 = Select(t="Try to reset the UUT" ("string"), s=w628, f="Burn Successed.") -> (s? t:f=w631:string)
      n280 = Concatenate Strings(w638, "\r\n", w631) -> (→"Error List":string)
    }
  }
  n281 = local read "Drv"() -> (w46:u8)
  n282 = flat-sequence {
    tunnel: w50 -> [w672]
    tunnel: w46 -> [w671]
    tunnel: w18 -> [w670]
    tunnel: [w655] -> w19
    frame #0 {
      n283 = Split Number(x=u32 0) -> (hi(x)=w668:u16, lo(x)=w667:u16)
      n284 = Split Number(x=w667) -> (hi(x)=w662:u8, lo(x)=w661:u8)
      n285 = Split Number(x=w668) -> (hi(x)=w660:u8, lo(x)=w659:u8)
      n286 = Replace Array Subset(array=u8[] [0, 0, 0, 0, 0, 0, 0, 0] ("unsigned byte array"), new element #1=w661, index #1=0 ("index"), new element #2=w662, new element #3=w659, new element #4=w660) -> (w663:u8[])  [unwired: 3 in]
      n287 = Byte Array To String(unsigned byte array=w663) -> (string=w657:string)
      n288 = call "TCPSend (SubVI).vi"("Opcode"=u32 4112, "error in"=w672, "string"=w657, "Drv"=w671, "connection ID"=w670) -> ("error out"=w669:errorcluster)  [unwired: 6 in]
      n289 = property on="stop Listen" class="Bool (strict)"(error in=w669, "Value"=TRUE ("stop Listen")) -> (error out=w655:errorcluster)  [unwired: 1 in, 1 out]
    }
  }
  n290 = call <vilib>:"Clear Errors.vi"("error in (no error)"=w19) -> ("error out"=w15:errorcluster)  [unwired: 5 in, 1 out]
  n291 = call "TCP_NoDelay_Windows.vi"("error in (no error)"=w15, "TCP_NODELAY (true)"=FALSE, "connID"=w18) -> ("error out"=w2:errorcluster, "connID 2"=w3:refnum<k5>)  [unwired: 3 in]
  n292 = call <vilib>:"Clear Errors.vi"("error in (no error)"=w2) -> ("error out"=w1:errorcluster)  [unwired: 5 in, 1 out]
  n293 = TCP Close Connection(connection ID=w3, error in (no error)=w1) -> (error out=→"error out":errorcluster)  [unwired: 1 in, 1 out]
